vi "nom,prénom.vi"() -> ()   [LabVIEW 2018]
panel:
  in  "Nom brut":string
  out "Boolean":bool
  out "Nom":string
  out "Prénom":string
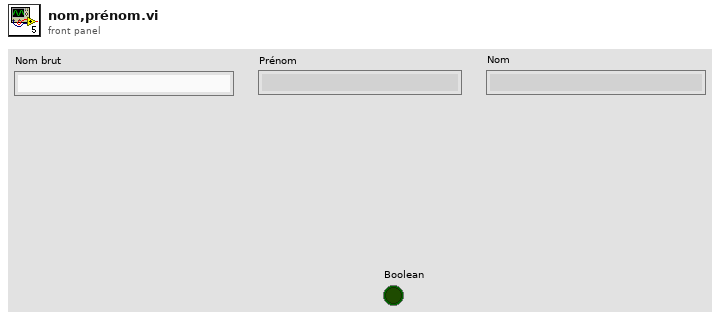
[diagram p1: front panel]
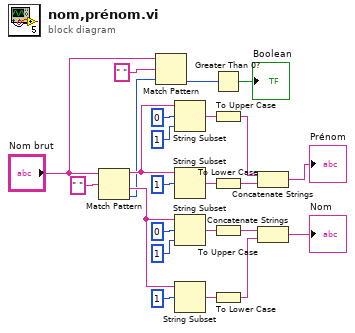
[diagram p0: block diagram]
diagram:
  n1 = Match Pattern(string="Nom brut", regular expression=" ") -> (before substring=w20:string, after substring=w14:string, offset past match=w1:i32)  [unwired: 1 in, 1 out]
  n2 = Match Pattern(string="Nom brut", regular expression=" ", offset (0)=w1) -> (offset past match=w3:i32)  [unwired: 3 out]
  n3 = String Subset(string=w20, offset (0)=0, length (rest)=1 ("length (rest)")) -> (substring=w19:string)
  n4 = String Subset(string=w20, offset (0)=1) -> (substring=w12:string)  [unwired: 1 in]
  n5 = String Subset(string=w14, offset (0)=0, length (rest)=1 ("length (rest)")) -> (substring=w10:string)
  n6 = String Subset(string=w14, offset (0)=1) -> (substring=w9:string)  [unwired: 1 in]
  n7 = Greater Than 0?(x=w3) -> (x > 0?=→"Boolean":bool)
  n8 = To Upper Case(1:w19) -> (0:w18:string)
  n9 = To Lower Case(string=w12) -> (all lower case string=w11:string)
  n10 = To Upper Case(1:w10) -> (0:w8:string)
  n11 = To Lower Case(string=w9) -> (all lower case string=w2:string)
  n12 = Concatenate Strings(w18, w11) -> (→"Prénom":string)
  n13 = Concatenate Strings(w8, w2) -> (→"Nom":string)
